vi "SPI Init.vi"(8 "Error In":errorcluster, 11 "ChipKit Resource":T1={"COM Port"="", "Board Type"=enum."ChipKit uC32", "Connection Type"=enum."USB / Serial", "Baud Rate (115200)"=15, "Bytes Per Packet (15)"=15, "DI Port Num Pins"=0, "DO Port Num Pins"=0}) -> (0 "Error Out":errorcluster, 3 "ChipKit Resource":T1={"COM Port"="", "Board Type"=enum."ChipKit uC32", "Connection Type"=enum."USB / Serial", "Baud Rate (115200)"=15, "Bytes Per Packet (15)"=15, "DI Port Num Pins"=0, "DO Port Num Pins"=0})   [LabVIEW 2011, in "LabVIEW Interface for ChipKit.lvlib"]
doc: "Initialize the SPI bus. \n\nChipkit uC32: SS Pin 10\n MOSI Pin 11 \n MISO Pin 12\n SCK Pin 13"
uses:
  LabVIEW Interface for ChipKit.lvlib
  Private/Type Defs/Chipkit Resource.ctl
  Private/Type Defs/Board Type.ctl
  Private/Type Defs/Connection Type.ctl
  Private/Type Defs/Command.ctl
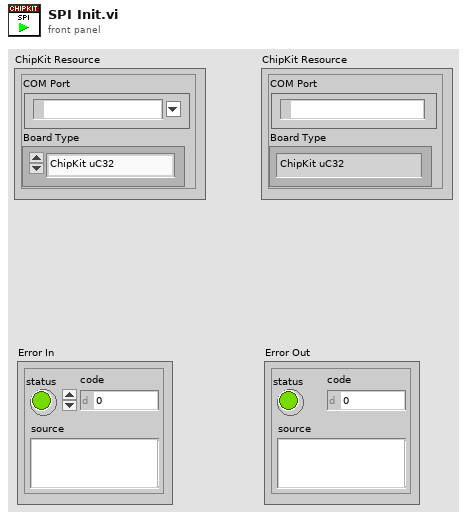
[diagram p1: front panel]
types:
  T1 = typedef "LabVIEW Interface for ChipKit.lvlib/Chipkit Resource.ctl" = cluster{"COM Port":refnum<visa-resource-name>, "Board Type":T2, "Connection Type":T3, "Baud Rate (115200)":u32, "Bytes Per Packet (15)":u32, "DI Port Num Pins":i32, "DO Port Num Pins":i32}
  T2 = typedef "LabVIEW Interface for ChipKit.lvlib/Board Type.ctl" = enum16{"ChipKit uC32", "ChipKit Uno32", "ChipKit Max32"}
  T3 = typedef "LabVIEW Interface for ChipKit.lvlib/Connection Type.ctl" = enum8{"USB / Serial", "XBEE", "BlueSmirf (Bluetooth)"}
  T4 = typedef "LabVIEW Interface for ChipKit.lvlib/Command.ctl" = enum8{"setArduinoMode", "flushSerial", "setPinMode", "digitalWritePin", "digitalWritePort", "tone", "digitalReadPin", "digitalReadPort", "analogReadPin", "analogReadPort", "pwmWritePin", "pwmWritePort", "sevenSegment_Configure", "sevenSegment_Write", "I2C Init", "I2C Write", "I2C Read", "SPI Init", "SPI Set Bit Order", "SPI Set Clock Divider", "SPI Set Data Mode", "SPI Send / Receive", "SPI Close", "Servo Set Num Servos", "Servo Config Servo", "Servo Write Angle", "Servo Read Angle", "Servo Write Pulse Width", "Servo Read Pulse Width", "Servo Detach", "LCD Init", "LCD Set Size", "LCD Set Cursor Mode", "LCD Clear", "LCD Set Cursor Position", "LCD Print", "LCD Display Power", "LCD Scroll Display", "LCD Autoscroll", "LCD Print Direction", "LCD Create Custom Char", "LCD Print Custom Char", "contAcqOn", "contAcqOff", "getFirmwareVersion", "FiniteSampleStart", "NA", "NA2", "Conifg Stepper", "Stepper Write", "Stepper Detach", "Stepper Steps To Go", "Config DO Port", "Config DI Port"}
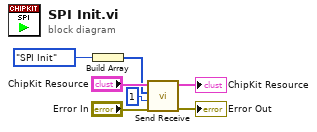
[diagram p0: block diagram]
diagram:
  n1 = Build Array(Command."SPI Init" ("Command")) -> (w5:T4[])
  n2 = call "Send Receive.vi"("Error In"="Error In", "Bytes To Read (0)"=u32 1, "Data"=w5, "ChipKit Resource"="ChipKit Resource") -> ("Error Out"=→"Error Out":errorcluster, "ChipKit Resource"=→"ChipKit Resource":T1)  [unwired: 5 in, 1 out]
